vi "ArmSetOverride.vi"(11 "Override":bool) -> ()   [LabVIEW 2023]
uses:
  ArmGlobal.vi
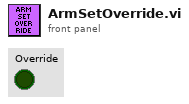
[diagram p1: front panel]
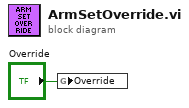
[diagram p0: block diagram]
diagram:
  n1 = global write "ArmGlobal.vi" "Override"("Override") -> ()
